vi "Add LED Backplane.vi"(8 "error in (no error)":errorcluster, 10 "Rack #":u8, 11 "Node Ptr":u64 format="%.0x") -> (0 "error out":errorcluster)   [LabVIEW 2014, in "SLSC configuration System Explorer.lvlib"]
uses:
  SLSC configuration System Explorer.lvlib
  Type Defs/Card Position.ctl
  Shared/SPI Utility/Slot #.ctl
  Shared/Constants.vi
  Shared/SLSC configuration Shared.lvlib
  <vilib>/NI Veristand/Custom Device API/Custom Device API.lvlib
panel:
  in  "Tag":string
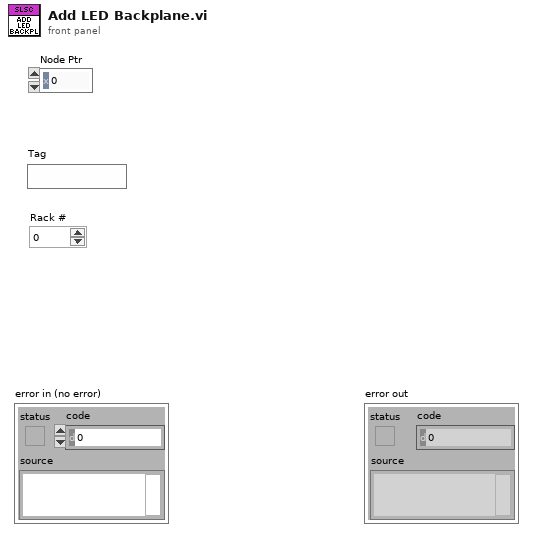
[diagram p1: front panel]
types:
  T1 = typedef "SLSC configuration Shared.lvlib/Card Position.ctl" = cluster{"Rack #":u8, "Slot #":T2}
  T2 = typedef "SLSC configuration Shared.lvlib/Slot #.ctl" = u8
  T3 = typedef "Custom Device API.lvlib/Custom Device Item Ref.ctl" = u64
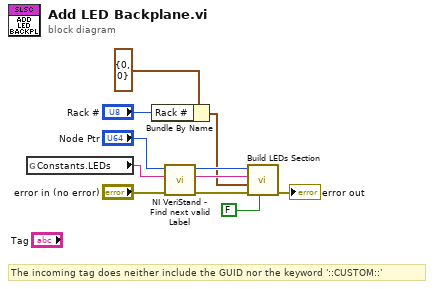
[diagram p0: block diagram]
diagram:
  # "The incoming tag does neither include the GUID nor the keyword '::CUSTOM::'"
  n1 = global read "Constants.vi" "Constants.LEDs"() -> (w9:string)
  n2 = Bundle By Name(cluster=T1 {"Rack #"=0, "Slot #"=0} ("Card Position"), "Rack #"="Rack #") -> (w2:T1)
  n3 = call <vilib>:"NI VeriStand - Find next valid Label.vi"("error in (no error)"="error in (no error)", "Label"=w9, "Item Ref in"="Node Ptr") -> ("error out"=w8:errorcluster, "Label out"=w6:string, "Item Ref out"=w5:T3)  [unwired: 4 in, 2 out]
  n4 = call "Build LEDs Section.vi"("Cancelled?"=FALSE, "error in (no error)"=w8, "Card Position in"=w2, "Name in"=w6, "Node Ptr in"=w5) -> ("error out"=→"error out":errorcluster)  [unwired: 6 in]
